vi "CRYUnflatten Curve Library.vi"(11 "Flatten CurLib":string) -> (0 "Error?":bool=TRUE, 2 "CurLib Cluster":T1 {"Waveforms"."Y dB ref" format="%.1f"; "Waveforms"."Y axis" items=["Log", "Lin"]; "Waveforms"."Y data" items=["dB", "Lin"]; "Waveforms"."X data" items=["dB", "Lin"]; "Values"."Z data" items=["dB", "Lin"]; "Values"."X data" items=["dB", "Lin"]; "Values"."Y data" items=["dB", "Lin"]; "Values"."Z dB ref" format="%.1f"; "Values"."Z axis" items=["Log", "Lin"]; "Values"."X dB ref" format="%.1f"; "Values"."X axis" items=["Log", "Lin"]; "Values"."Y axis" items=["Log", "Lin"]; "Values"."Y dB ref" format="%.1f"; "Values"."Curve"."z" format="%.2f"; "Values"."Curve"."y" format="%.2f"; "Values"."Curve"."x" format="%.2f"; "Results"."Margin" format="%.2f"; "Curves"."Z data" items=["dB", "Lin"]; "Curves"."X data" items=["dB", "Lin"]; "Curves"."Y data" items=["dB", "Lin"]; "Curves"."Z dB ref" format="%.1f"; "Curves"."Z axis" items=["Log", "Lin"]; "Curves"."X dB ref" format="%.1f"; "Curves"."X axis" items=["Log", "Lin"]; "Curves"."Y axis" items=["Log", "Lin"]; "Curves"."Y dB ref" format="%.1f"; "Curves"."Curve"."z" format="%.2f"; "Curves"."Curve"."y" format="%.2f"; "Curves"."Curve"."x" format="%.2f"}, 3 "Header info":T8={"Data type"="Data            ", "Version"=1, "Dimensions"=0})   [LabVIEW 2013]
uses:
  Control/CRYCurve Library Cluster.ctl
  CRYSystem/Typedef Control/CRYData Cluster Array.ctl
  CRYSystem/Typedef Control/CRYData Cluster.ctl
  CRYSystem/Typedef Control/CRYResult Cluster Array.ctl
  CRYSystem/Typedef Control/CRYResult Cluster.ctl
  CRYSystem/Typedef Control/CRYWaveform Cluster Array.ctl
  CRYSystem/Typedef Control/CRYWaveform Cluster.ctl
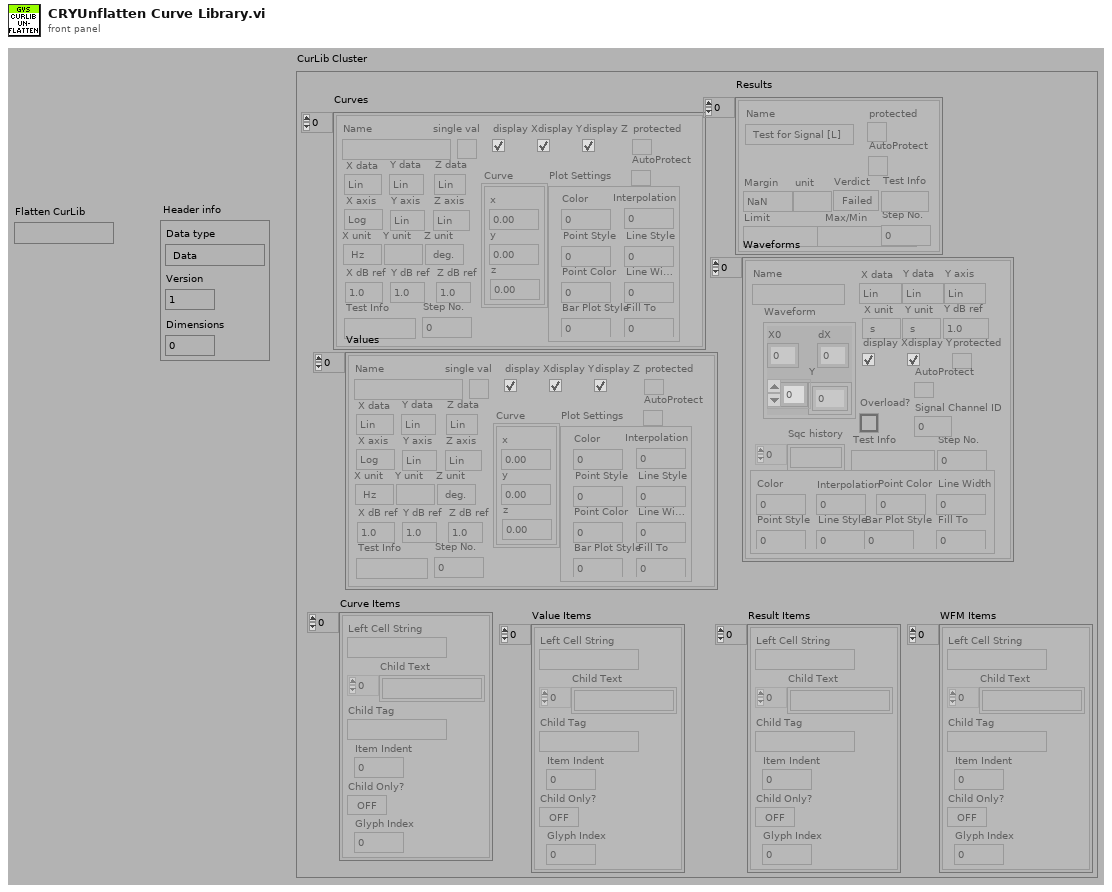
[diagram p1: front panel]
types:
  T1 = typedef "CRYCurve Library Cluster.ctl" = cluster{"Curves":T2, "Results":T4, "Values":T2, "Waveforms":T6, "Curve Items":cluster{"Left Cell String":string, "Child Text":string[], "Child Tag":string, "Item Indent":i32, "Child Only?":bool, "Glyph Index":i32}[], "Value Items":cluster{"Left Cell String":string, "Child Text":string[], "Child Tag":string, "Item Indent":i32, "Child Only?":bool, "Glyph Index":i32}[], "Result Items":cluster{"Left Cell String":string, "Child Text":string[], "Child Tag":string, "Item Indent":i32, "Child Only?":bool, "Glyph Index":i32}[], "WFM Items":cluster{"Left Cell String":string, "Child Text":string[], "Child Tag":string, "Item Indent":i32, "Child Only?":bool, "Glyph Index":i32}[]}
  T2 = typedef "CRYData Cluster Array.ctl" = T3[]
  T3 = typedef "CRYData Cluster.ctl" = cluster{"Name":string, "Curve":cluster{"x":dbl, "y":dbl, "z":dbl}[], "X data":u16, "Y data":u16, "Z data":u16, "X axis":u16, "Y axis":u16, "Z axis":u16, "X unit":string, "Y unit":string, "Z unit":string, "X dB ref":dbl, "Y dB ref":dbl, "Z dB ref":dbl, "single val":bool, "protected":bool, "display X":bool, "display Y":bool, "display Z":bool, "Test Info":string, "Step No.":i32, "Plot Settings":cluster{"Color":u32, "Interpolation":u8, "Point Style":u8, "Line Style":u8, "Point Color":u32, "Line Width":u8, "Bar Plot Style":u8, "Fill To":i16}, "AutoProtect":bool}
  T4 = typedef "CRYResult Cluster Array.ctl" = T5[]
  T5 = typedef "CRYResult Cluster.ctl" = cluster{"Name":string, "Margin":dbl, "unit":string, "Verdict":bool, "Limit":string, "Max/Min":string, "protected":bool, "Step No.":i32, "Test Info":string, "AutoProtect":bool}
  T6 = typedef "CRYWaveform Cluster Array.ctl" = T7[]
  T7 = typedef "CRYWaveform Cluster.ctl" = cluster{"Waveform":cluster{"X0":dbl, "dX":dbl, "Y":sgl[]}, "X data":u16, "Y data":u16, "Y axis":u16, "X unit":string, "Y unit":string, "Y dB ref":dbl, "display Y":bool, "display X":bool, "Overload?":bool, "Test Info":string, "Step No.":i32, "Name":string, "protected":bool, "Sqc history":string[], "Signal Channel ID":i32, "Plot Settings":cluster{"Color":u32, "Interpolation":u8, "Point Style":u8, "Line Style":u8, "Point Color":u32, "Line Width":u8, "Bar Plot Style":u8, "Fill To":i16}, "AutoProtect":bool}
  T8 = cluster{"Data type":string, "Version":u16, "Dimensions":u8}
  T9 = cluster{"Curves":T2, "Results":T4, "Values":T2, "Waveforms":T6, "Curve Items":cluster{"Left Cell String":string, "Child Text":string[], "Child Tag":string, "Item Indent":i32, "Child Only?":bool, "Glyph Index":i32}[], "Value Items":cluster{"Left Cell String":string, "Child Text":string[], "Child Tag":string, "Item Indent":i32, "Child Only?":bool, "Glyph Index":i32}[], "Result Items":cluster{"Left Cell String":string, "Child Text":string[], "Child Tag":string, "Item Indent":i32, "Child Only?":bool, "Glyph Index":i32}[], "WFM Items":cluster{"Left Cell String":string, "Child Text":string[], "Child Tag":string, "Item Indent":i32, "Child Only?":bool, "Glyph Index":i32}[]}
  T10 = cluster{"unsigned byte array[0]":u8, "unsigned byte array[1]":u8, "unsigned byte array[2]":u8}
  T11 = cluster{"Curves":cluster{"Name":string, "Curve":cluster{"x":dbl, "y":dbl, "z":dbl}[], "X data":u16, "Y data":u16, "Z data":u16, "X axis":u16, "Y axis":u16, "Z axis":u16, "X unit":string, "Y unit":string, "Z unit":string, "X dB ref":dbl, "Y dB ref":dbl, "Z dB ref":dbl, "single val":bool, "protected":bool, "display X":bool, "display Y":bool, "display Z":bool, "Test Info":string, "Step No.":u16, "Plot Settings":cluster{"Color":u32, "Interpolation":u8, "Point Style":u8, "Line Style":u8, "Point Color":u32, "Line Width":u8, "Bar Plot Style":u8, "Fill To":i16}, "AutoProtect":bool}[], "Results":cluster{"Name":string, "Margin":dbl, "unit":string, "Verdict":bool, "Limit":string, "Max/Min":string, "protected":bool, "Step No.":u16, "Test Info":string, "AutoProtect":bool}[], "Values":cluster{"Name":string, "Curve":cluster{"x":dbl, "y":dbl, "z":dbl}[], "X data":u16, "Y data":u16, "Z data":u16, "X axis":u16, "Y axis":u16, "Z axis":u16, "X unit":string, "Y unit":string, "Z unit":string, "X dB ref":dbl, "Y dB ref":dbl, "Z dB ref":dbl, "single val":bool, "protected":bool, "display X":bool, "display Y":bool, "display Z":bool, "Test Info":string, "Step No.":u16, "Plot Settings":cluster{"Color":u32, "Interpolation":u8, "Point Style":u8, "Line Style":u8, "Point Color":u32, "Line Width":u8, "Bar Plot Style":u8, "Fill To":i16}, "AutoProtect":bool}[], "Waveforms":cluster{"Waveform":cluster{"X0":dbl, "dX":dbl, "Y":sgl[]}, "X data":u16, "Y data":u16, "Y axis":u16, "X unit":string, "Y unit":string, "Y dB ref":dbl, "display Y":bool, "display X":bool, "Overload?":bool, "Test Info":string, "Step No.":u16, "Name":string, "protected":bool, "Sqc history":string[], "Signal Channel ID":i32, "Plot Settings":cluster{"Color":u32, "Interpolation":u8, "Point Style":u8, "Line Style":u8, "Point Color":u32, "Line Width":u8, "Bar Plot Style":u8, "Fill To":i16}, "AutoProtect":bool}[]}
  T12 = cluster{"Name":string, "Curve":cluster{"x":dbl, "y":dbl, "z":dbl}[], "X data":u16, "Y data":u16, "Z data":u16, "X axis":u16, "Y axis":u16, "Z axis":u16, "X unit":string, "Y unit":string, "Z unit":string, "X dB ref":dbl, "Y dB ref":dbl, "Z dB ref":dbl, "single val":bool, "protected":bool, "display X":bool, "display Y":bool, "display Z":bool, "Test Info":string, "Step No.":u16, "Plot Settings":cluster{"Color":u32, "Interpolation":u8, "Point Style":u8, "Line Style":u8, "Point Color":u32, "Line Width":u8, "Bar Plot Style":u8, "Fill To":i16}, "AutoProtect":bool}[]
  T13 = cluster{"Name":string, "Margin":dbl, "unit":string, "Verdict":bool, "Limit":string, "Max/Min":string, "protected":bool, "Step No.":u16, "Test Info":string, "AutoProtect":bool}[]
  T14 = cluster{"Waveform":cluster{"X0":dbl, "dX":dbl, "Y":sgl[]}, "X data":u16, "Y data":u16, "Y axis":u16, "X unit":string, "Y unit":string, "Y dB ref":dbl, "display Y":bool, "display X":bool, "Overload?":bool, "Test Info":string, "Step No.":u16, "Name":string, "protected":bool, "Sqc history":string[], "Signal Channel ID":i32, "Plot Settings":cluster{"Color":u32, "Interpolation":u8, "Point Style":u8, "Line Style":u8, "Point Color":u32, "Line Width":u8, "Bar Plot Style":u8, "Fill To":i16}, "AutoProtect":bool}[]
  T15 = cluster{"Color":u32, "Interpolation":u8, "Point Style":u8, "Line Style":u8, "Point Color":u32, "Line Width":u8, "Bar Plot Style":u8, "Fill To":i16}
  T16 = cluster{"Curves":T2, "Results":T4, "Values":T2, "Waveforms":T6}
  T17 = cluster{"Left Cell String":string, "Child Text":string[], "Child Tag":string, "Item Indent":i32, "Child Only?":bool, "Glyph Index":i32}
  T18 = cluster{"Left Cell String":string, "Child Text":string[], "Child Tag":string, "Item Indent":i32, "Child Only?":bool, "Glyph Index":i32}[]
  T19 = cluster{"substring":string, u16, "unsigned byte array[2]":u8}
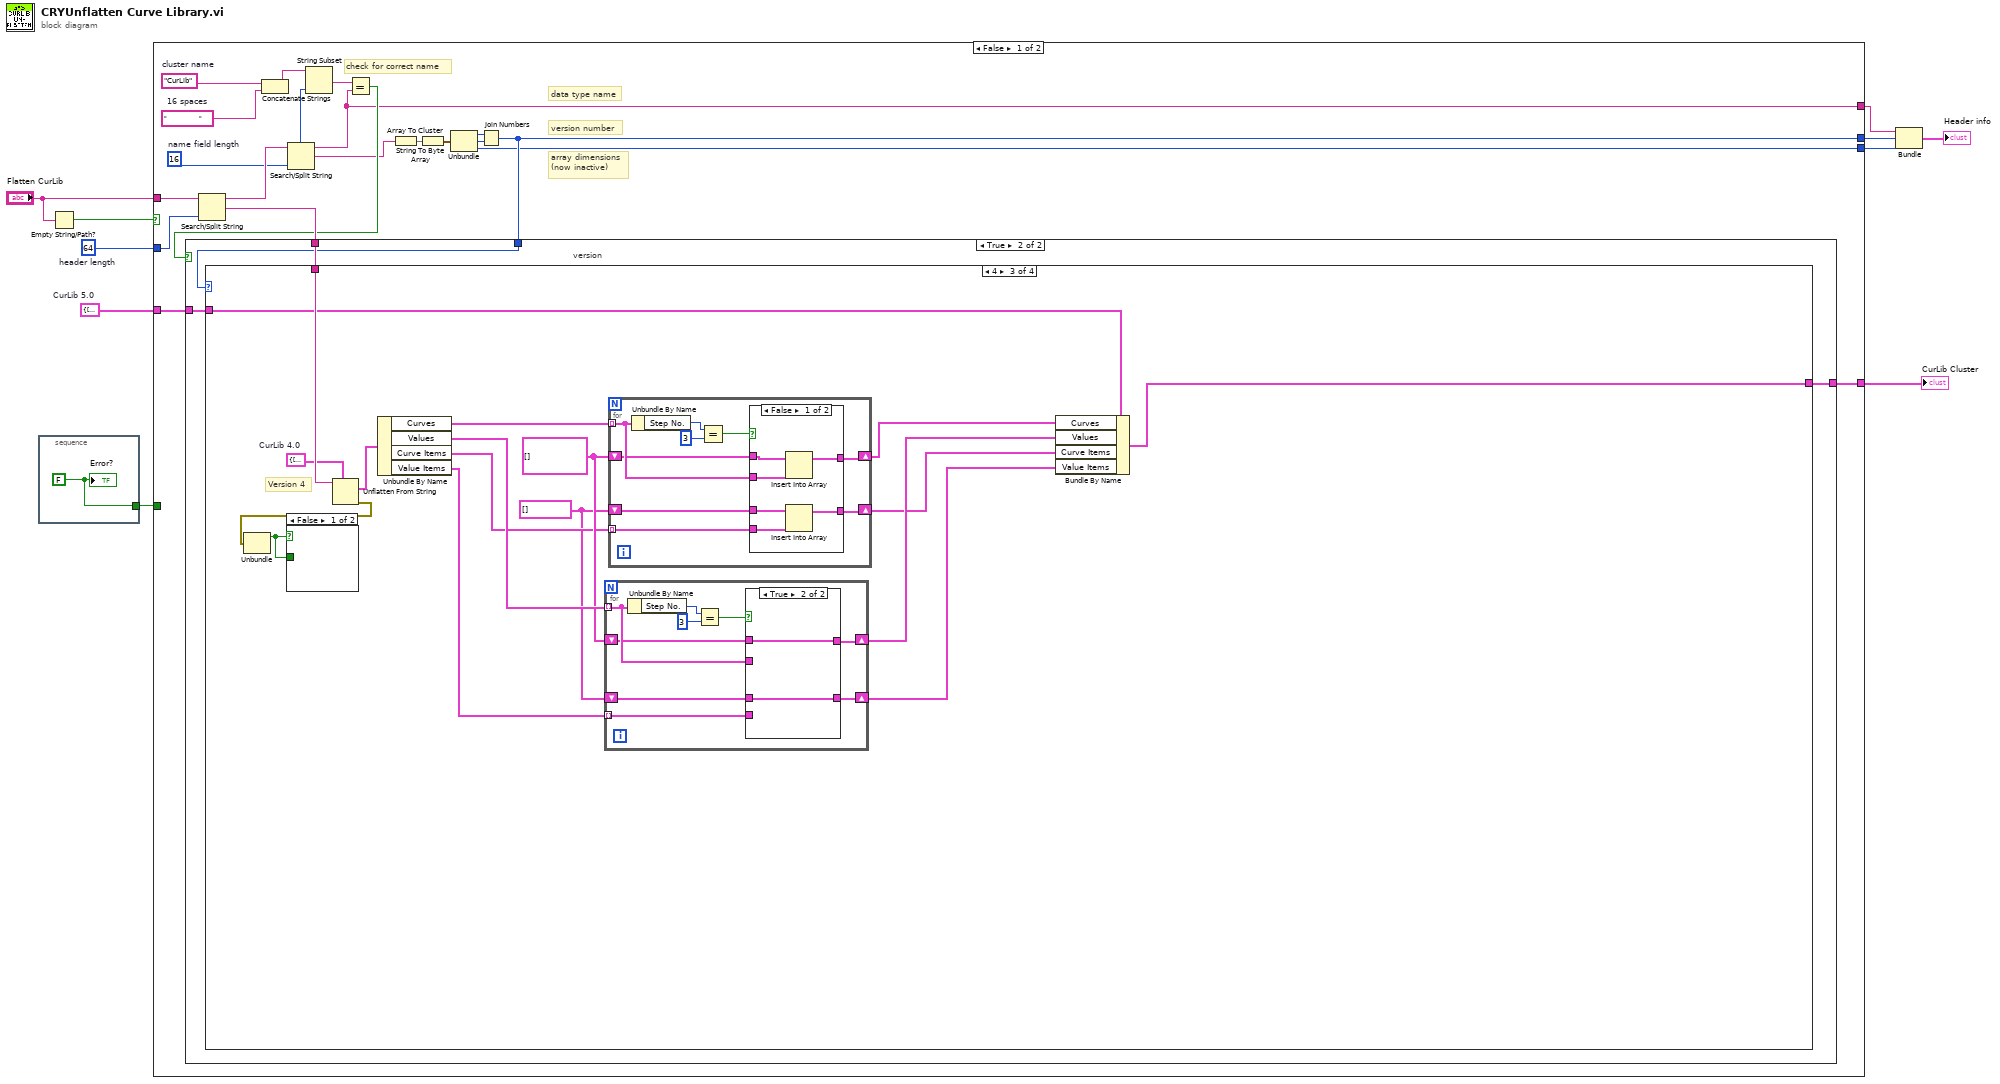
[diagram p0: block diagram]
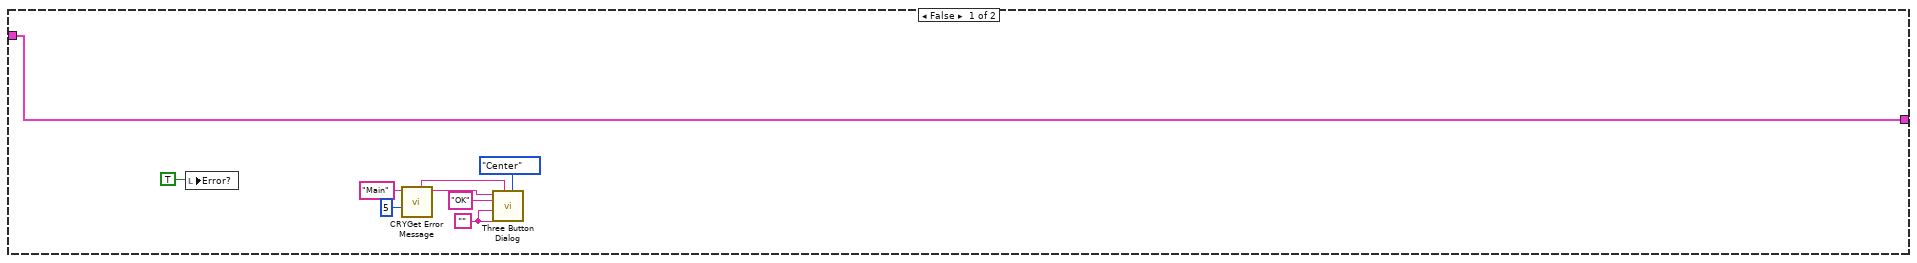
[diagram p2: hidden frame]
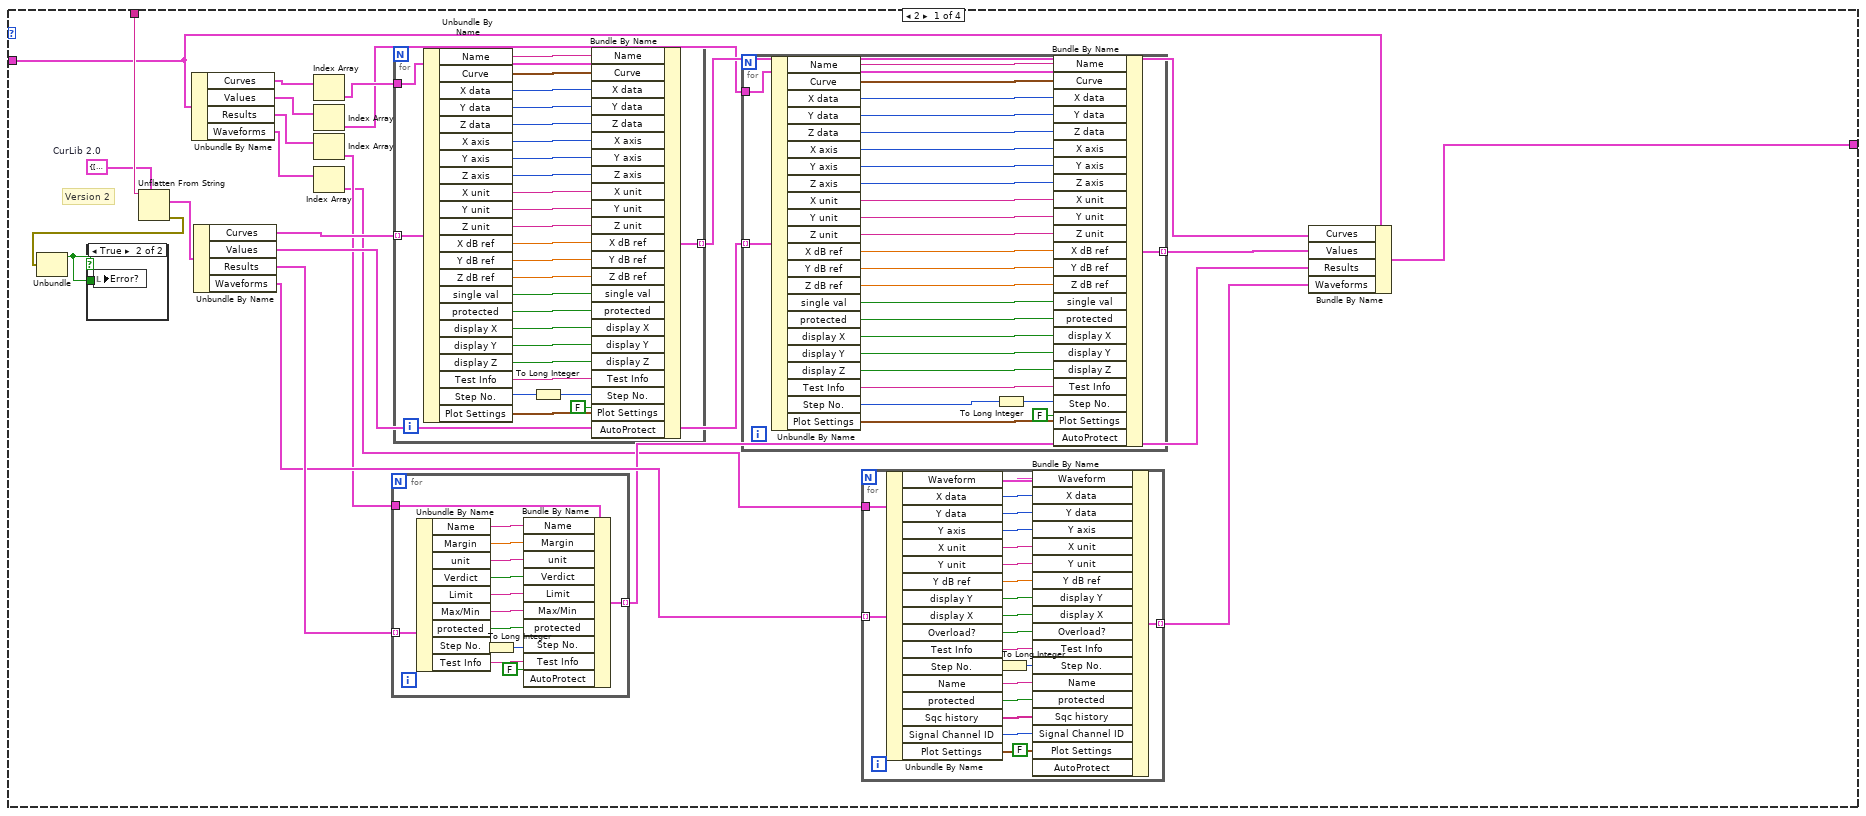
[diagram p3: hidden frame]
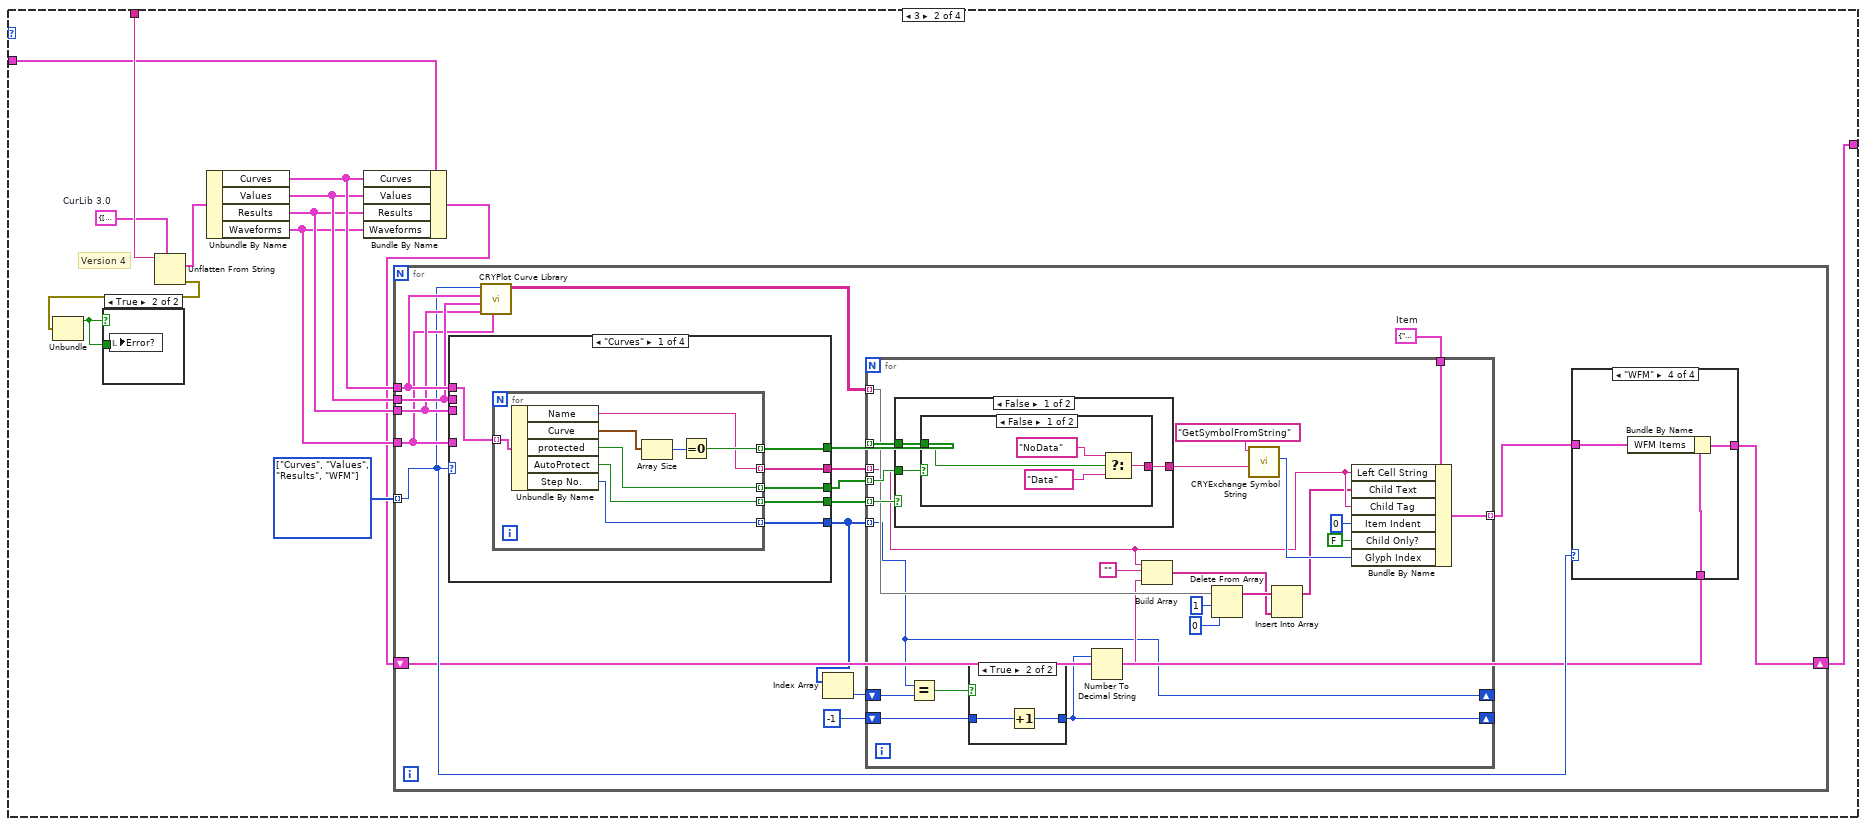
[diagram p5: hidden frame]
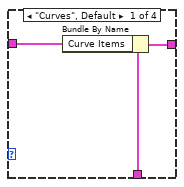
[diagram p6: hidden frame]
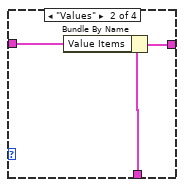
[diagram p7: hidden frame]
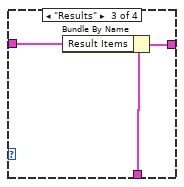
[diagram p8: hidden frame]
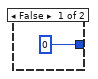
[diagram p9: hidden frame]
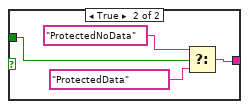
[diagram p10: hidden frame]
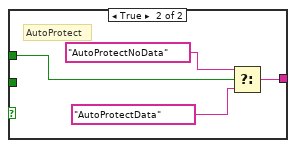
[diagram p11: hidden frame]
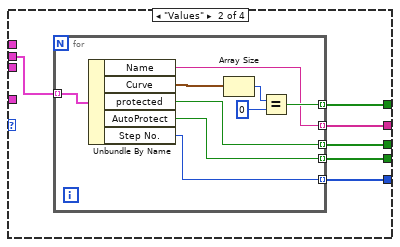
[diagram p12: hidden frame]
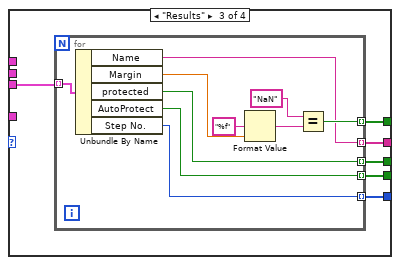
[diagram p13: hidden frame]
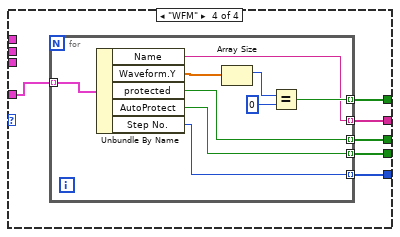
[diagram p14: hidden frame]
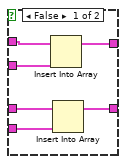
[diagram p16: hidden frame]
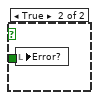
[diagram p18: hidden frame]
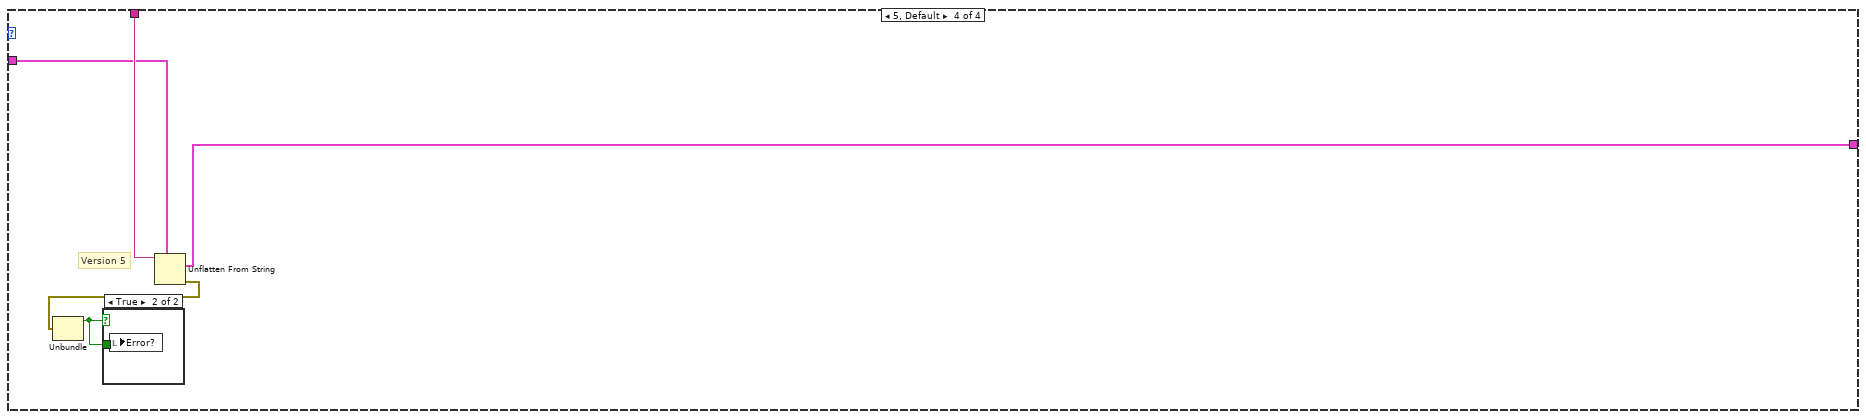
[diagram p19: hidden frame]
diagram:
  w2 = T9 {"Curves"=[], "Results"=[], "Values"=[], "Waveforms"=[], "Curve Items"=[], "Value Items"=[], "Result Items"=[], "WFM Items"=[]}  # CurLib 5.0
  w8 = 64  # header length
  n1 = stacked-sequence {
    tunnel: [w11] -> w3
    frame #0 {
      w11 = FALSE
      "Error?" <- w11
    }
  }
  n2 = Empty String/Path?(string/path="Flatten CurLib") -> (empty?=w9:bool)
  n3 = case shown="False" w9 {
    tunnel: "Flatten CurLib" -> [w31 _]
    tunnel: w8 -> [w25 _]
    tunnel: [w22 u16 0] -> w6
    tunnel: [w14 u8 0] -> w7
    tunnel: [w15 "(no data input)" ("substring")] -> w5
    tunnel: w3 -> [_ _]
    tunnel: [w13 w362] -> w1
    tunnel: w2 -> [w12 w362]
    frame False {
      w19 = "                "  # 16 spaces
      w20 = "CurLib"  # cluster name
      w17 = 16  # name field length
      # "check for correct name"
      # "array dimensions\n(now inactive)"
      # "version number"
      # "data type name"
      n4 = Search/Split String(string=w31, offset (0)=w25) -> (substring before match=w24:string, match + rest of string=w26:string)  [unwired: 2 out]
      n5 = Concatenate Strings(w20, w19) -> (w18:string)
      n6 = Search/Split String(string=w24, offset (0)=w17) -> (substring before match=w15:string, match + rest of string=w21:string)  [unwired: 2 out]
      n7 = String Subset(string=w18, length (rest)=w17) -> (substring=w16:string)  [unwired: 1 out]
      n8 = Equal?(x=w16, y=w15) -> (x = y?=w23:bool)
      n9 = String To Byte Array(string=w21) -> (unsigned byte array=w30:u8[])
      n10 = Array To Cluster(array=w30) -> (cluster=w29:T10)
      n11 = Unbundle(w29) -> ("unsigned byte array[0]"=w28:u8, "unsigned byte array[1]"=w27:u8, "unsigned byte array[2]"=w14:u8)
      n12 = Join Numbers(hi=w28, lo=w27) -> ((hi.lo)=w22:u16)
      n13 = case shown="True" w23 {
        tunnel: w26 -> [_ w44]
        tunnel: w22 -> [_ w43]
        tunnel: [w32 w42] -> w13
        tunnel: w12 -> [w32 w41]
        frame False {
          w39 = ""
          n14 = local write "Error?"(TRUE) -> ()
          n15 = call "CRYGet Error Message.vi"("Error No"=5, "Kind"="Main") -> ("Message"=w34:string, "Window Title"=w33:string)  [unwired: 4 in, 4 out]
          n16 = call <vilib>:"Three Button Dialog.vi"("Justify Message (Left)"=enum16{"Left", "Center", "Right"}."Center", "Window Title (\"\")"=w33, "Right Button Text (\"Cancel\")"=w39, "Center Button Text (\"No\")"=w39, "Left Button Text (\"Yes\")"="OK" ("Left Button Text (\"Yes\")"), "message"=w34) -> ()  [unwired: 6 out]
        }
        frame True {
          n17 = case "version" shown="4" w43 {
            tunnel: w44 -> [w67 w171 w320 w360]
            tunnel: [w63 w159 w312 w357] -> w42
            tunnel: w41 -> [w46 w167 w304 w356]
            frame 2 {
              w45 = T11 {"Curves"=[], "Results"=[], "Values"=[], "Waveforms"=[]}  # CurLib 2.0
              # "Version 2"
              n18 = Unflatten From String(type=w45, binary string=w67) -> (value=w64:T11, error out=w65:errorcluster)  [unwired: 1 in, 3 out]
              n19 = Unbundle(w65) -> ("status"=w66:bool)  [unwired: 2 out]
              n20 = case shown="True" w66 {
                tunnel: w66 -> [_ w158]
                frame False {
                }
                frame True {
                  n21 = local write "Error?"(w158) -> ()
                }
              }
              n22 = Unbundle By Name(w46) -> ("Curves"=w54:T2, "Values"=w52:T2, "Results"=w50:T4, "Waveforms"=w48:T6)
              n23 = Unbundle By Name(w64) -> ("Curves"=w62:T12, "Values"=w60:T12, "Results"=w58:T13, "Waveforms"=w57:T14)
              n24 = Index Array(array=w54) -> (element=w53:T3)  [unwired: 1 in]
              n25 = Index Array(array=w52) -> (element=w51:T3)  [unwired: 1 in]
              n26 = Index Array(array=w50) -> (element=w49:T5)  [unwired: 1 in]
              n27 = Index Array(array=w48) -> (element=w47:T7)  [unwired: 1 in]
              n28 = for {
                tunnel: w49 -> [w102]
                tunnel: w58 -> [w103] mode=indexing
                tunnel: [w91] -> w55 mode=indexing
                n29 = Unbundle By Name(w103) -> ("Name"=w101:string, "Margin"=w100:dbl, "unit"=w98:string, "Verdict"=w99:bool, "Limit"=w96:string, "Max/Min"=w97:string, "protected"=w95:bool, "Step No."=w94:u16, "Test Info"=w93:string)
                n30 = To Long Integer(number=w94) -> (32bit integer=w90:i32)
                n31 = Bundle By Name(cluster=w102, "Name"=w101, "Margin"=w100, "unit"=w98, "Verdict"=w99, "Limit"=w96, "Max/Min"=w97, "protected"=w95, "Step No."=w90, "Test Info"=w93, "AutoProtect"=FALSE) -> (w91:T5)
              }
              n32 = for {
                tunnel: w62 -> [w157] mode=indexing
                tunnel: w53 -> [w156]
                tunnel: [w155] -> w61 mode=indexing
                n33 = Unbundle By Name(w157) -> ("Name"=w154:string, "Curve"=w153:cluster{"x":dbl, "y":dbl, "z":dbl}[], "X data"=w152:u16, "Y data"=w151:u16, "Z data"=w150:u16, "X axis"=w149:u16, "Y axis"=w148:u16, "Z axis"=w147:u16, "X unit"=w146:string, "Y unit"=w145:string, "Z unit"=w144:string, "X dB ref"=w143:dbl, "Y dB ref"=w142:dbl, "Z dB ref"=w141:dbl, "single val"=w140:bool, "protected"=w139:bool, "display X"=w138:bool, "display Y"=w137:bool, "display Z"=w136:bool, "Test Info"=w135:string, "Step No."=w134:u16, "Plot Settings"=w133:T15)
                n34 = To Long Integer(number=w134) -> (32bit integer=w131:i32)
                n35 = Bundle By Name(cluster=w156, "Name"=w154, "Curve"=w153, "X data"=w152, "Y data"=w151, "Z data"=w150, "X axis"=w149, "Y axis"=w148, "Z axis"=w147, "X unit"=w146, "Y unit"=w145, "Z unit"=w144, "X dB ref"=w143, "Y dB ref"=w142, "Z dB ref"=w141, "single val"=w140, "protected"=w139, "display X"=w138, "display Y"=w137, "display Z"=w136, "Test Info"=w135, "Step No."=w131, "Plot Settings"=w133, "AutoProtect"=FALSE) -> (w155:T3)
              }
              n36 = for {
                tunnel: w60 -> [w130] mode=indexing
                tunnel: w51 -> [w129]
                tunnel: [w128] -> w59 mode=indexing
                n37 = Unbundle By Name(w130) -> ("Name"=w127:string, "Curve"=w126:cluster{"x":dbl, "y":dbl, "z":dbl}[], "X data"=w125:u16, "Y data"=w124:u16, "Z data"=w123:u16, "X axis"=w122:u16, "Y axis"=w121:u16, "Z axis"=w120:u16, "X unit"=w119:string, "Y unit"=w118:string, "Z unit"=w117:string, "X dB ref"=w116:dbl, "Y dB ref"=w115:dbl, "Z dB ref"=w114:dbl, "single val"=w113:bool, "protected"=w112:bool, "display X"=w111:bool, "display Y"=w110:bool, "display Z"=w109:bool, "Test Info"=w108:string, "Step No."=w107:u16, "Plot Settings"=w106:T15)
                n38 = To Long Integer(number=w107) -> (32bit integer=w104:i32)
                n39 = Bundle By Name(cluster=w129, "Name"=w127, "Curve"=w126, "X data"=w125, "Y data"=w124, "Z data"=w123, "X axis"=w122, "Y axis"=w121, "Z axis"=w120, "X unit"=w119, "Y unit"=w118, "Z unit"=w117, "X dB ref"=w116, "Y dB ref"=w115, "Z dB ref"=w114, "single val"=w113, "protected"=w112, "display X"=w111, "display Y"=w110, "display Z"=w109, "Test Info"=w108, "Step No."=w104, "Plot Settings"=w106, "AutoProtect"=FALSE) -> (w128:T3)
              }
              n40 = for {
                tunnel: w47 -> [w88]
                tunnel: w57 -> [w89] mode=indexing
                tunnel: [w69] -> w56 mode=indexing
                n41 = Unbundle By Name(w89) -> ("Waveform"=w87:cluster{"X0":dbl, "dX":dbl, "Y":sgl[]}, "X data"=w86:u16, "Y data"=w85:u16, "Y axis"=w84:u16, "X unit"=w83:string, "Y unit"=w82:string, "Y dB ref"=w81:dbl, "display Y"=w80:bool, "display X"=w79:bool, "Overload?"=w78:bool, "Test Info"=w77:string, "Step No."=w76:u16, "Name"=w75:string, "protected"=w74:bool, "Sqc history"=w73:string[], "Signal Channel ID"=w72:i32, "Plot Settings"=w71:T15)
                n42 = To Long Integer(number=w76) -> (32bit integer=w68:i32)
                n43 = Bundle By Name(cluster=w88, "Waveform"=w87, "X data"=w86, "Y data"=w85, "Y axis"=w84, "X unit"=w83, "Y unit"=w82, "Y dB ref"=w81, "display Y"=w80, "display X"=w79, "Overload?"=w78, "Test Info"=w77, "Step No."=w68, "Name"=w75, "protected"=w74, "Sqc history"=w73, "Signal Channel ID"=w72, "Plot Settings"=w71, "AutoProtect"=FALSE) -> (w69:T7)
              }
              n44 = Bundle By Name(cluster=w46, "Curves"=w61, "Values"=w59, "Results"=w55, "Waveforms"=w56) -> (w63:T9)
            }
            frame 3 {
              w161 = enum16{"Curves", "Values", "Results", "WFM"}[] [enum."Curves", enum."Values", enum."Results", enum."WFM"] items=["Curves", "Values", "Results", "WFM"]
              w168 = T16 {"Curves"=[], "Results"=[], "Values"=[], "Waveforms"=[]}  # CurLib 3.0
              # "Version 4"
              n45 = Unflatten From String(type=w168, binary string=w171) -> (value=w166:T16, error out=w169:errorcluster)  [unwired: 1 in, 3 out]
              n46 = Unbundle(w169) -> ("status"=w170:bool)  [unwired: 2 out]
              n47 = case shown="True" w170 {
                tunnel: w170 -> [_ w303]
                frame False {
                }
                frame True {
                  n48 = local write "Error?"(w303) -> ()
                }
              }
              n49 = Unbundle By Name(w166) -> ("Curves"=w165:T2, "Values"=w164:T2, "Results"=w163:T4, "Waveforms"=w162:T6)
              n50 = Bundle By Name(cluster=w167, "Curves"=w165, "Values"=w164, "Results"=w163, "Waveforms"=w162) -> (w160:T9)
              n51 = for {
                tunnel: w165 -> [w188]
                tunnel: w164 -> [w187]
                tunnel: w163 -> [w186]
                tunnel: w162 -> [w185]
                tunnel: w161 -> [w178] mode=indexing
                shift-right: [w176] -> w159
                shift-left: w160 -> [w177]
                w180 = T17 {"Left Cell String"="", "Child Text"=[], "Child Tag"="", "Item Indent"=0, "Child Only?"=FALSE, "Glyph Index"=0}  # Item
                n52 = case shown="\"Curves\"" w178 {
                  tunnel: [w248 w262 w277 w293] -> w184
                  tunnel: [w247 w261 w276 w292] -> w179
                  tunnel: [w246 w260 w275 w291] -> w183
                  tunnel: [w245 w259 w274 w290] -> w182
                  tunnel: w188 -> [w244 _ _ _]
                  tunnel: w187 -> [_ w258 _ _]
                  tunnel: w186 -> [_ _ w273 _]
                  tunnel: w185 -> [_ _ _ w289]
                  tunnel: [w243 w257 w272 w288] -> w173
                  frame "Curves" {
                    n53 = for {
                      tunnel: w244 -> [w255] mode=indexing
                      tunnel: [w254] -> w248 mode=indexing
                      tunnel: [w250] -> w247 mode=indexing
                      tunnel: [w252] -> w246 mode=indexing
                      tunnel: [w251] -> w245 mode=indexing
                      tunnel: [w249] -> w243 mode=indexing
                      n54 = Unbundle By Name(w255) -> ("Name"=w250:string, "Curve"=w256:cluster{"x":dbl, "y":dbl, "z":dbl}[], "protected"=w252:bool, "AutoProtect"=w251:bool, "Step No."=w249:i32)
                      n55 = Array Size(array=w256) -> (size(s)=w253:i32)
                      n56 = Equal To 0?(x=w253) -> (x = 0?=w254:bool)
                    }
                  }
                  frame "Values" {
                    n57 = for {
                      tunnel: w258 -> [w270] mode=indexing
                      tunnel: [w267] -> w262 mode=indexing
                      tunnel: [w264] -> w261 mode=indexing
                      tunnel: [w266] -> w260 mode=indexing
                      tunnel: [w265] -> w259 mode=indexing
                      tunnel: [w263] -> w257 mode=indexing
                      n58 = Unbundle By Name(w270) -> ("Name"=w264:string, "Curve"=w271:cluster{"x":dbl, "y":dbl, "z":dbl}[], "protected"=w266:bool, "AutoProtect"=w265:bool, "Step No."=w263:i32)
                      n59 = Array Size(array=w271) -> (size(s)=w268:i32)
                      n60 = Equal?(x=w268, y=0) -> (x = y?=w267:bool)
                    }
                  }
                  frame "Results" {
                    n61 = for {
                      tunnel: w273 -> [w287] mode=indexing
                      tunnel: [w286] -> w277 mode=indexing
                      tunnel: [w279] -> w276 mode=indexing
                      tunnel: [w281] -> w275 mode=indexing
                      tunnel: [w280] -> w274 mode=indexing
                      tunnel: [w278] -> w272 mode=indexing
                      n62 = Unbundle By Name(w287) -> ("Name"=w279:string, "Margin"=w285:dbl, "protected"=w281:bool, "AutoProtect"=w280:bool, "Step No."=w278:i32)
                      n63 = Format Value(format string="%f", value (0)=w285) -> (output string=w282:string)  [unwired: 1 in]
                      n64 = Equal?(x="NaN", y=w282) -> (x = y?=w286:bool)
                    }
                  }
                  frame "WFM" {
                    n65 = for {
                      tunnel: w289 -> [w299] mode=indexing
                      tunnel: [w298] -> w293 mode=indexing
                      tunnel: [w295] -> w292 mode=indexing
                      tunnel: [w297] -> w291 mode=indexing
                      tunnel: [w296] -> w290 mode=indexing
                      tunnel: [w294] -> w288 mode=indexing
                      n66 = Unbundle By Name(w299) -> ("Name"=w295:string, "Waveform.Y"=w301:sgl[], "protected"=w297:bool, "AutoProtect"=w296:bool, "Step No."=w294:i32)
                      n67 = Array Size(array=w301) -> (size(s)=w302:i32)
                      n68 = Equal?(x=w302, y=0) -> (x = y?=w298:bool)
                    }
                  }
                }
                n69 = call "CRYPlot Curve Library.vi"("Waveform"=w185, "Results"=w186, "Values"=w187, "Curves"=w188, "Type"=w178) -> ("PlotStrings"=w181:string[][])  [unwired: 6 in]
                n70 = Index Array(array=w173) -> (element=w172:i32)  [unwired: 1 in]
                n71 = for {
                  tunnel: w184 -> [w224] mode=indexing
                  tunnel: w183 -> [w223] mode=indexing
                  tunnel: w182 -> [w222] mode=indexing
                  tunnel: w181 -> [w216] mode=indexing
                  tunnel: w180 -> [w219]
                  tunnel: w179 -> [w211] mode=indexing
                  tunnel: [w212] -> w175 mode=indexing
                  tunnel: w173 -> [w203] mode=indexing
                  shift-right: [w204] -> _
                  shift-left: -1 ("Step No.") -> [w206]
                  shift-right: [w203] -> _
                  shift-left: w172 -> [w208]
                  n72 = case shown="False" w222 {
                    tunnel: w224 -> [w229 w242]
                    tunnel: [w228 w241] -> w220
                    tunnel: w223 -> [w230 _]
                    frame False {
                      n73 = case shown="False" w230 {
                        tunnel: w229 -> [w234 w238]
                        tunnel: [w233 w237] -> w228
                        frame False {
                          n74 = Select(t="NoData" ("name or relative path"), s=w234, f="Data" ("name or relative path")) -> (s? t:f=w233:string)
                        }
                        frame True {
                          n75 = Select(t="ProtectedNoData" ("name or relative path"), s=w238, f="ProtectedData" ("name or relative path")) -> (s? t:f=w237:string)
                        }
                      }
                    }
                    frame True {
                      # "AutoProtect"
                      n76 = Select(t="AutoProtectNoData" ("name or relative path"), s=w242, f="AutoProtectData" ("name or relative path")) -> (s? t:f=w241:string)
                    }
                  }
                  n77 = Equal?(x=w203, y=w208) -> (x = y?=w207:bool)
                  n78 = case shown="True" w207 {
                    tunnel: w206 -> [_ w227]
                    tunnel: [0 ("Step No.") w226] -> w204
                    frame False {
                    }
                    frame True {
                      n79 = Increment(x=w227) -> (x+1=w226:i32)
                    }
                  }
                  n80 = Number To Decimal String(number=w204) -> (decimal integer string=w205:string)  [unwired: 1 in]
                  n81 = Build Array(w211, "", w205) -> (w209:string[])
                  n82 = Delete From Array(array=w216, length=1, index=0) -> (array with subset deleted=w210:string[])  [unwired: 1 out]
                  n83 = call "CRYExchange Symbol String.vi"("sData"=w220, "sAction"="GetSymbolFromString") -> ("nData out"=w214:i32)  [unwired: 8 in, 1 out]
                  n84 = Insert Into Array(array=w210, new element=w209) -> (w202:string[])  [unwired: 1 in]
                  n85 = Bundle By Name(cluster=w219, "Left Cell String"=w211, "Child Text"=w202, "Child Tag"=w211, "Item Indent"=0, "Child Only?"=FALSE, "Glyph Index"=w214) -> (w212:T17)
                }
                n86 = case shown="\"WFM\"" w178 {
                  tunnel: w177 -> [w191 w194 w197 w200]
                  tunnel: [w190 w193 w196 w199] -> w176
                  tunnel: w175 -> [w189 w192 w195 w198]
                  frame "Curves", Default {
                    n87 = Bundle By Name(cluster=w191, "Curve Items"=w189) -> (w190:T9)
                  }
                  frame "Values" {
                    n88 = Bundle By Name(cluster=w194, "Value Items"=w192) -> (w193:T9)
                  }
                  frame "Results" {
                    n89 = Bundle By Name(cluster=w197, "Result Items"=w195) -> (w196:T9)
                  }
                  frame "WFM" {
                    n90 = Bundle By Name(cluster=w200, "WFM Items"=w198) -> (w199:T9)
                  }
                }
              }
            }
            frame 4 {
              w305 = T9 {"Curves"=[], "Results"=[], "Values"=[], "Waveforms"=[], "Curve Items"=[], "Value Items"=[], "Result Items"=[], "WFM Items"=[]}  # CurLib 4.0
              w309 = T18 [] ("Curve Items")
              w311 = T2 [] ("Curves")
              # "Version 4"
              n91 = Unflatten From String(type=w305, binary string=w320) -> (value=w317:T9, error out=w318:errorcluster)  [unwired: 1 in, 3 out]
              n92 = Unbundle(w318) -> ("status"=w319:bool)  [unwired: 2 out]
              n93 = case shown="False" w319 {
                tunnel: w319 -> [_ w355]
                frame False {
                }
                frame True {
                  n94 = local write "Error?"(w355) -> ()
                }
              }
              n95 = Unbundle By Name(w317) -> ("Curves"=w316:T2, "Values"=w313:T2, "Curve Items"=w310:T18, "Value Items"=w308:T18)
              n96 = for {
                tunnel: w313 -> [w327] mode=indexing
                shift-right: [w324] -> w314
                shift-left: w311 -> [w325]
                shift-right: [w322] -> w306
                shift-left: w309 -> [w323]
                tunnel: w308 -> [w321] mode=indexing
                n97 = Unbundle By Name(w327) -> ("Step No."=w329:i32)
                n98 = Equal?(x=w329, y=3) -> (x = y?=w326:bool)
                n99 = case shown="True" w326 {
                  tunnel: w327 -> [w333 _]
                  tunnel: w325 -> [w335 w337]
                  tunnel: [w334 w337] -> w324
                  tunnel: w323 -> [w332 w336]
                  tunnel: [w331 w336] -> w322
                  tunnel: w321 -> [w330 _]
                  frame False {
                    n100 = Insert Into Array(array=w335, new element=w333) -> (w334:T2)  [unwired: 1 in]
                    n101 = Insert Into Array(array=w332, new element=w330) -> (w331:T18)  [unwired: 1 in]
                  }
                  frame True {
                  }
                }
              }
              n102 = for {
                tunnel: w316 -> [w344] mode=indexing
                shift-right: [w341] -> w315
                shift-left: w311 -> [w342]
                shift-right: [w339] -> w307
                shift-left: w309 -> [w340]
                tunnel: w310 -> [w338] mode=indexing
                n103 = Unbundle By Name(w344) -> ("Step No."=w346:i32)
                n104 = Equal?(x=w346, y=3) -> (x = y?=w343:bool)
                n105 = case shown="False" w343 {
                  tunnel: w344 -> [w350 _]
                  tunnel: w342 -> [w352 w354]
                  tunnel: [w351 w354] -> w341
                  tunnel: w340 -> [w349 w353]
                  tunnel: [w348 w353] -> w339
                  tunnel: w338 -> [w347 _]
                  frame False {
                    n106 = Insert Into Array(array=w352, new element=w350) -> (w351:T2)  [unwired: 1 in]
                    n107 = Insert Into Array(array=w349, new element=w347) -> (w348:T18)  [unwired: 1 in]
                  }
                  frame True {
                  }
                }
              }
              n108 = Bundle By Name(cluster=w304, "Curves"=w315, "Values"=w314, "Curve Items"=w307, "Value Items"=w306) -> (w312:T9)
            }
            frame 5, Default {
              # "Version 5"
              n109 = Unflatten From String(type=w356, binary string=w360) -> (value=w357:T9, error out=w358:errorcluster)  [unwired: 1 in, 3 out]
              n110 = Unbundle(w358) -> ("status"=w359:bool)  [unwired: 2 out]
              n111 = case shown="True" w359 {
                tunnel: w359 -> [_ w361]
                frame False {
                }
                frame True {
                  n112 = local write "Error?"(w361) -> ()
                }
              }
            }
          }
        }
      }
    }
    frame True {
      n113 = local write "Error?"(TRUE ("Error?")) -> ()
    }
  }
  "CurLib Cluster" <- w1
  n114 = Bundle("substring"=w5, w6, "unsigned byte array[2]"=w7) -> (→"Header info":T19)  [unwired: 1 out]
